vi "FileIO_MoveFileAndRenameWithTimeStamp.vi"(0 "Source Path":path, 5 "Target Path":path, 11 "Error In":errorcluster) -> (4 "New Path":path, 15 "Error Out":errorcluster)   [LabVIEW 2016]
doc: "This VI will move a file from one directory to another with a new file name which includes the Date/Time stamp in file name. It does not copy the file, therefore file will only be in new location."
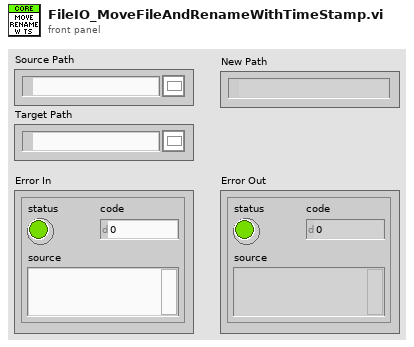
[diagram p1: front panel]
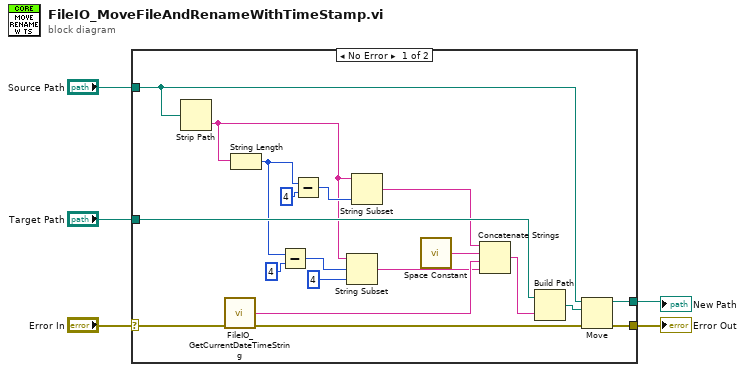
[diagram p0: block diagram]
diagram:
  n1 = case shown="No Error" "Error In" {
    selector: "Error In" -> [w24 w25]
    tunnel: "Target Path" -> [w16 _]
    tunnel: [w19 w25] -> w4
    tunnel: "Source Path" -> [w6 _]
    tunnel: [w18 _] -> w1
    frame No Error {
      n2 = Strip Path(path=w6) -> (name=w9:string)  [unwired: 1 out]
      n3 = call "FileIO_GetCurrentDateTimeString.vi"("Error In"=w24) -> ("Date/Time String"=w21:string, "Error Out"=w23:errorcluster)  [unwired: 13 in]
      n4 = String Length(string=w9) -> (length=w7:i32)
      n5 = Subtract(x=w7, y=4) -> (x-y=w14:i32)
      n6 = Subtract(x=w7, y=4) -> (x-y=w11:i32)
      n7 = String Subset(string=w9, offset (0)=w14, length (rest)=4 ("length (rest)")) -> (substring=w12:string)
      n8 = String Subset(string=w9, length (rest)=w11) -> (substring=w8:string)  [unwired: 1 in]
      n9 = call <vilib>:"Space Constant.vi"() -> ("String"=w22:string)
      n10 = Concatenate Strings(w8, w22, w21, w12) -> (w20:string)
      n11 = Build Path(base path=w16, name or relative path=w20) -> (appended path=w17:path)
      n12 = Move(source path=w6, error in=w23, 10:w17) -> (error out=w19:errorcluster, 3:w18:path)  [unwired: 2 in, 1 out]
    }
    frame Error {
    }
  }
  "Error Out" <- w4
  "New Path" <- w1
